vi "QueryAxisMotorType.vi"(8 "error in (no error)":errorcluster, 11 "Picomoto8742ControllerClass in":refnum<class "Picomoto8742ControllerClass.lvclass">) -> (0 "error out":errorcluster, 3 "Picomoto8742ControllerClass out":refnum<class "Picomoto8742ControllerClass.lvclass">)   [LabVIEW 2020, in "Picomoto8742ControllerClass.lvclass"]
doc: "Query the motor type setting, relative to the active axis, from the physical device"
uses:
  Picomoto8742ControllerClass.lvclass
  Picomoto8742ControllerClass.lvclass/Picomoto8742ControllerClass.ctl
  PicoMotor8742Axis/Picomotor8742Axis.lvclass
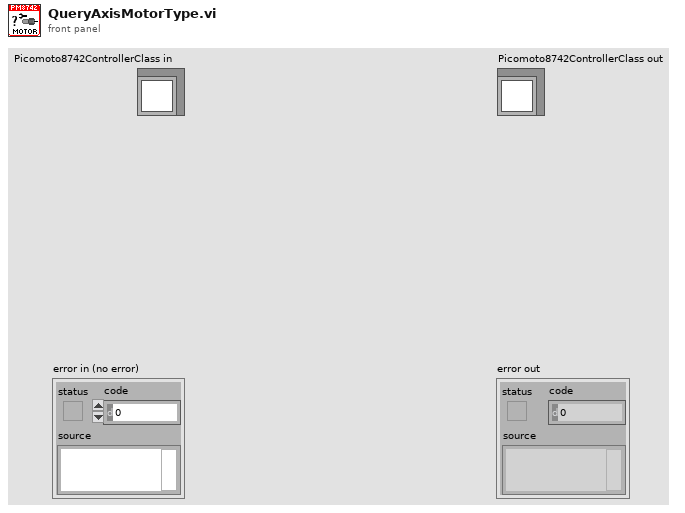
[diagram p1: front panel]
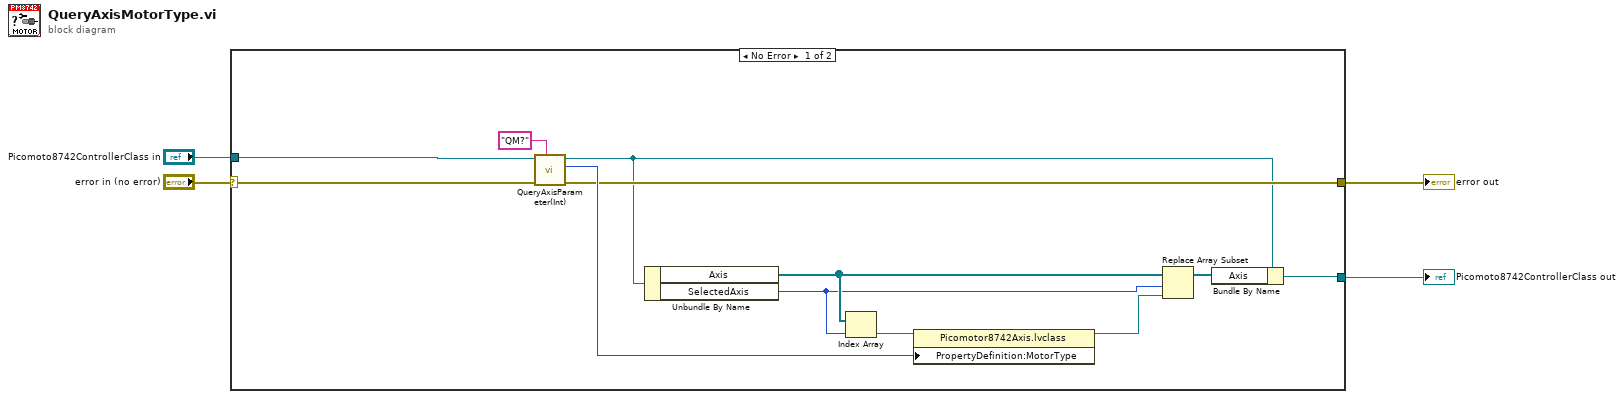
[diagram p0: block diagram]
diagram:
  n1 = case shown="No Error" "error in (no error)" {
    selector: "error in (no error)" -> [w6 w18]
    tunnel: [w15 w18] -> w3
    tunnel: [w12 w17] -> w1
    tunnel: "Picomoto8742ControllerClass in" -> [w5 w17]
    frame No Error {
      n2 = call-dynamic "QueryAxisParameter(Int).vi"("Cmd"="QM?" ("string"), "error in (no error)"=w6, "Picomoto8742ControllerClass in"=w5) -> ("error out"=w15:errorcluster, "ValueOut"=w16:i32, "Picomoto8742ControllerClass Out"=w7:refnum<class "Picomoto8742ControllerClass.lvclass">)  [unwired: 6 in]
      n3 = Unbundle By Name(w7) -> ("Axis"=w10:refnum<class "Picomotor8742Axis.lvclass">[], "SelectedAxis"=w9:u32)
      n4 = Index Array(array=w10, index=w9) -> (element=w8:refnum<class "Picomotor8742Axis.lvclass">)
      n5 = property class="Picomotor8742Axis.lvclass"(reference=w8, "PropertyDefinition:MotorType"=w16) -> (reference out=w14:refnum<class "Picomotor8742Axis.lvclass">)  [unwired: 1 in, 1 out]
      n6 = Replace Array Subset(array=w10, new element=w14, index=w9) -> (w13:refnum<class "Picomotor8742Axis.lvclass">[])
      n7 = Bundle By Name(cluster=w7, "Axis"=w13) -> (w12:refnum<class "Picomoto8742ControllerClass.lvclass">)
    }
    frame Error {
    }
  }
  "error out" <- w3
  "Picomoto8742ControllerClass out" <- w1
